vi "Method One Return Value.vi"(8 "error in (no error)":errorcluster, 11 "Test Interface Mock in":refnum<class "Test Interface Mock.lvclass">) -> (0 "error out":errorcluster, 2 "Return Value":dbl, 3 "Test Interface Mock out":refnum<class "Test Interface Mock.lvclass">)   [LabVIEW 2020, in "Test Interface Mock.lvclass"]
uses:
  Test Interface Mock.lvclass
  C:/git/astemes-lmock/source/Framework/Mock/Responsive Mock.lvclass
  source/Framework/Responsive Mock/Responsive Mock.lvclass
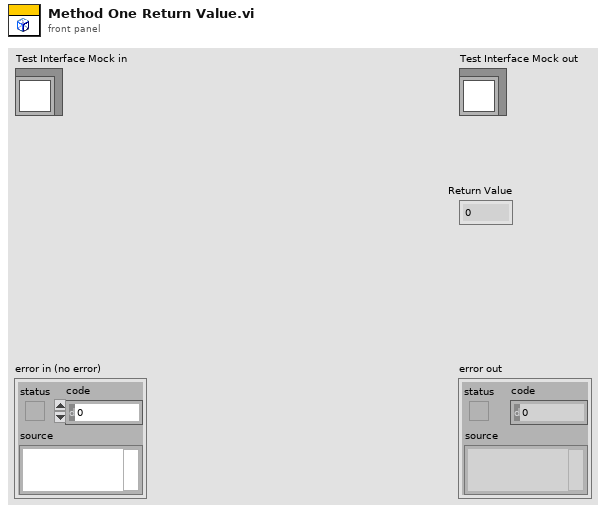
[diagram p1: front panel]
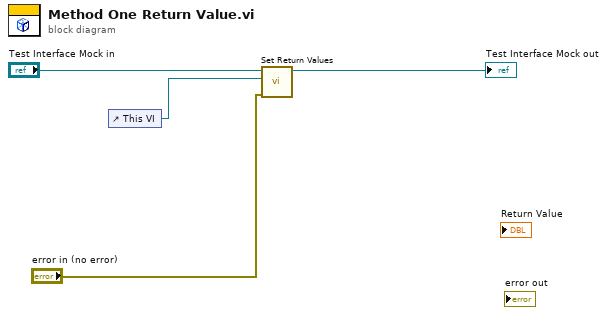
[diagram p0: block diagram]
diagram:
  n1 = control-ref of="This VI"() -> (w2:refnum<vi>)
  n2 = call "Set Return Values.vi"("error in (no error)"="error in (no error)", "VI Reference"=w2, "Mock In"="Test Interface Mock in") -> ("Mock Out"=→"Test Interface Mock out":refnum<class "Test Interface Mock.lvclass">)  [unwired: 7 in, 1 out]
